vi "CrawlingPrechargeState.vi"(8 "error in (no error)":errorcluster, 9 "Cluster in":T2, 10 "Enum in":T1, 11 "Actual Start [i]":i64) -> (0 "error out":errorcluster, 2 "Cluster out":T2, 3 "Enum":T1)   [LabVIEW 2018]
uses:
  Type_Def/Type_Def Actuator Controls.ctl
  Type_Def/Type_Def ControlState.ctl
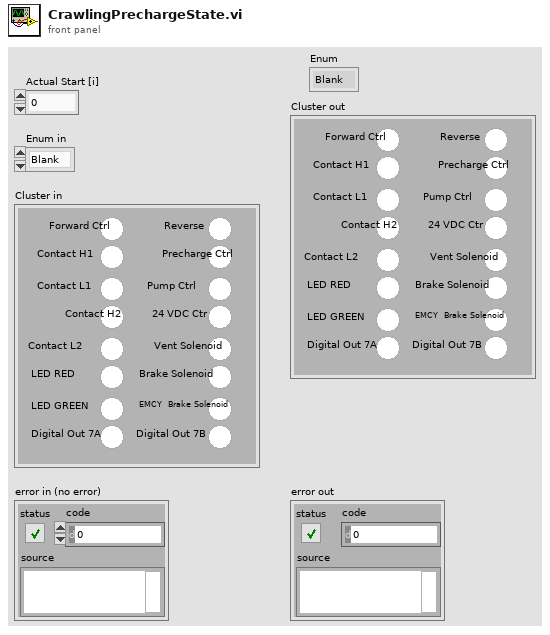
[diagram p1: front panel]
types:
  T1 = typedef "Type_Def ControlState.ctl" = enum16{"Blank", "Systems Check", "Idle", "Ready", "Pushing", "CrawlingPrecharge", "Braking", "Fault", "Boot Up", "Unpowered", "Crawling", "Shutdown", "Service Push", "Service Wait", "Vent", "Precharge"}
  T2 = typedef "Type_Def Actuator Controls.ctl" = cluster{"Reverse ":bool, "Precharge Ctrl":bool, "Pump Ctrl":bool, "24 VDC Ctr":bool, "Vent Solenoid":bool, "Brake Solenoid":bool, "EMCY  Brake Solenoid":bool, "Digital Out 7B ":bool, "Forward Ctrl":bool, "Contact H1":bool, "Contact L1":bool, "Contact H2":bool, "Contact L2 ":bool, "LED RED":bool, "LED GREEN":bool, " Digital Out 7A":bool}
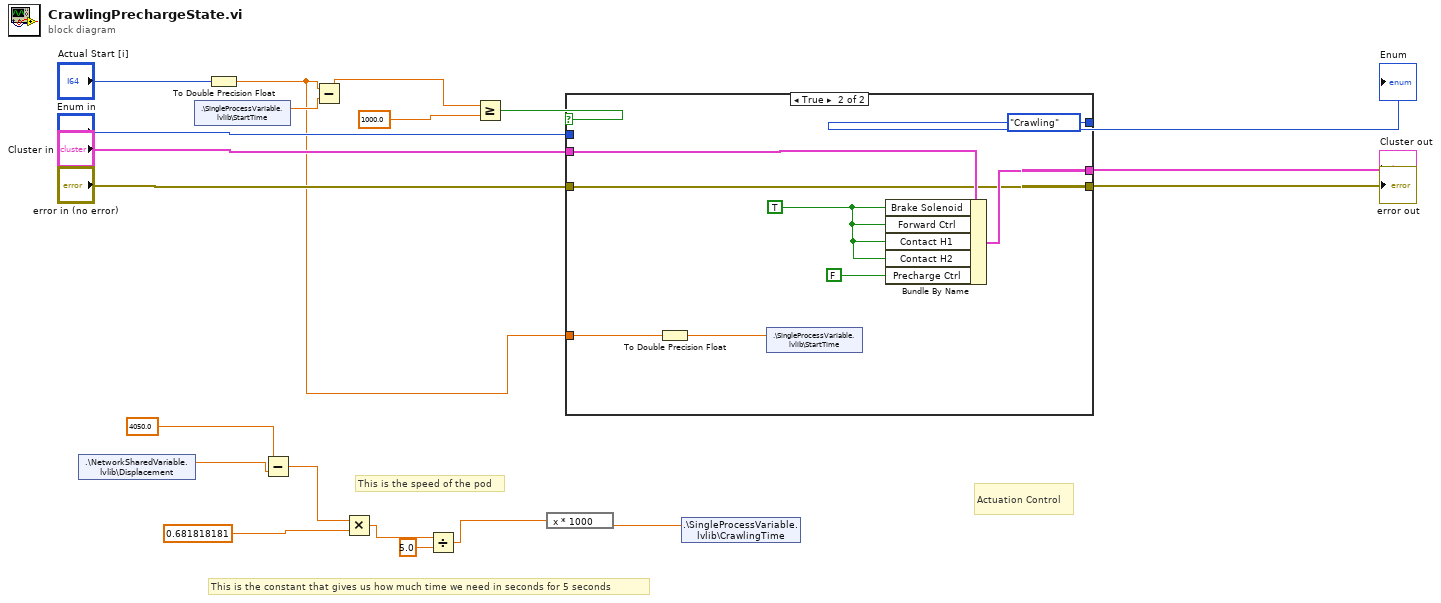
[diagram p0: block diagram]
diagram:
  # "This is the speed of the pod"
  # "This is the constant that gives us how much time we need in seconds for 5 seconds"
  # "Actuation Control"
  n1 = shared-variable ".\\NetworkSharedVariable.lvlib\\Displacement"() -> (w18:dbl)  [unwired: 1 in, 1 out]
  n2 = shared-variable ".\\SingleProcessVariable.lvlib\\StartTime"() -> (w12:dbl)  [unwired: 1 in, 1 out]
  n3 = To Double Precision Float(number="Actual Start [i]") -> (double precision float=w5:dbl)
  n4 = Subtract(x=4050.0, y=w18) -> (x-y=w19:dbl)
  n5 = Subtract(x=w5, y=w12) -> (x-y=w14:dbl)
  n6 = Multiply(x=w19, y=0.681818181) -> (x*y=w3:dbl)
  n7 = Divide(x=w3, y=5.0) -> (x/y=w1:dbl)
  n8 = Greater Or Equal?(x=w14, y=1000.0) -> (x >= y?=w16:bool)
  n9 = expression code="x * 1000"(w1) -> (w4:dbl)
  n10 = case shown="True" w16 {
    tunnel: "Enum in" -> [w23 _]
    tunnel: [w23 Type_Def_ControlState."Crawling"] -> w7
    tunnel: "Cluster in" -> [w22 w30]
    tunnel: [w22 w29] -> w9
    tunnel: [w21 w28] -> w10
    tunnel: "error in (no error)" -> [w21 w28]
    tunnel: w5 -> [_ w25]
    frame False {
    }
    frame True {
      w26 = TRUE ("Digital Out 5")
      n11 = To Double Precision Float(number=w25) -> (double precision float=w24:dbl)
      n12 = shared-variable ".\\SingleProcessVariable.lvlib\\StartTime"(w24) -> ()  [unwired: 1 in, 1 out]
      n13 = Bundle By Name(cluster=w30, "Brake Solenoid"=w26, "Forward Ctrl"=w26, "Contact H1"=w26, "Contact H2"=w26, "Precharge Ctrl"=FALSE ("Digital Out 5")) -> (w29:T2)
    }
  }
  "error out" <- w10
  "Cluster out" <- w9
  "Enum" <- w7
  n14 = shared-variable ".\\SingleProcessVariable.lvlib\\CrawlingTime"(w4) -> ()  [unwired: 1 in, 1 out]
